vi "close.vi"(8 "error in (no error)":errorcluster caption="错误输入（无错误）", 11 "WebDAV client 输入":refnum<class "WebDAV client.lvclass">) -> (0 "error out":errorcluster caption="错误输出", 3 "WebDAV client 输出":refnum<class "WebDAV client.lvclass">)   [LabVIEW 2016, in "数据传输系统.lvlib" / "update.lvlib" / "WebDAV client.lvclass"]
uses:
  WebDAV client.lvclass
  WebDAV client.lvclass/WebDAV client.ctl
  <vilib>/WebDAVClient/NI_WebDAV.lvlib
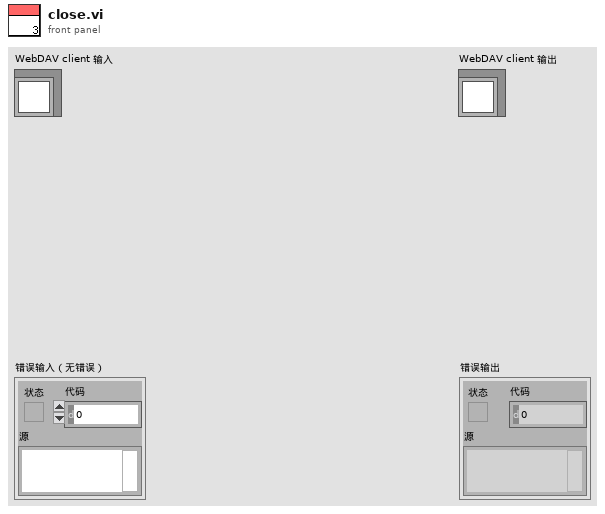
[diagram p1: front panel]
types:
  T1 = typedef "NI_WebDAV.lvlib/Asynchronous Session Handle.ctl" = refnum<k1>
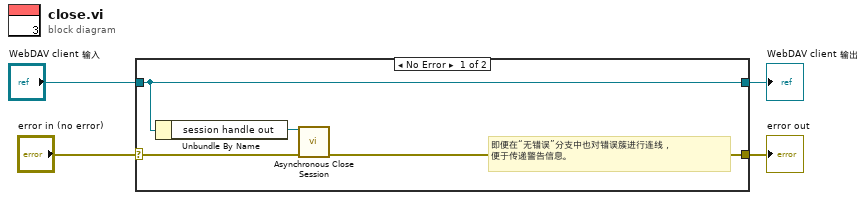
[diagram p0: block diagram]
diagram:
  n1 = case shown="No Error" "error in (no error)" {
    selector: "error in (no error)" -> [w6 w10]
    tunnel: [w5 w10] -> w3
    tunnel: [w8 w9] -> w1
    tunnel: "WebDAV client 输入" -> [w8 w9]
    frame No Error {
      # "即便在“无错误”分支中也对错误簇进行连线，\n便于传递警告信息。"
      n2 = Unbundle By Name(w8) -> ("session handle out"=w7:T1)
      n3 = call <vilib>:"Asynchronous Close Session.vi"("session handle"=w7, "error in (no error)"=w6) -> ("error out"=w5:errorcluster)  [unwired: 13 in]
    }
    frame Error {
    }
  }
  "error out" <- w3
  "WebDAV client 输出" <- w1
